vi "RX_RY.vi"(1 "RX/RY":string, 2 "Prg.no":string) -> (0 "RX-RY":string)   [LabVIEW 2024]
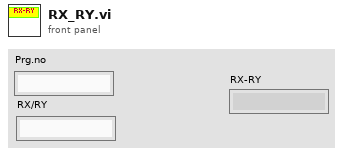
[diagram p1: front panel]
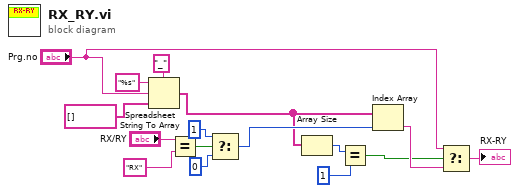
[diagram p0: block diagram]
diagram:
  n1 = Spreadsheet String To Array(delimiter (Tab)="_", format string="%s", spreadsheet string="Prg.no", array type (2D Dbl)=string[] [] ("y")) -> (array=w4:string[])
  n2 = Equal?(x="RX/RY", y="RX") -> (x = y?=w11:bool)
  n3 = Select(t=1 ("index"), s=w11, f=0 ("index")) -> (s? t:f=w8:i32)
  n4 = Array Size(array=w4) -> (size(s)=w3:i32)
  n5 = Equal?(x=w3, y=1) -> (x = y?=w1:bool)
  n6 = Index Array(array=w4, index=w8) -> (element=w6:string)
  n7 = Select(t="Prg.no", s=w1, f=w6) -> (s? t:f=→"RX-RY":string)
